vi "waypointVote.vi"() -> ()   [LabVIEW 2012]
panel:
  out "X of Center":dbl
  out "Y of Center":dbl
  out "XY Graph":cluster{dbl[], dbl[]}(graph)
  out "Radius":dbl
  in  "Boat Heading":dbl
  in  "Boat Pixel Y":dbl
  in  "Boat Pixel X":dbl
  in  "Desired Pixel Y":dbl
  in  "Desired Pixel X":dbl
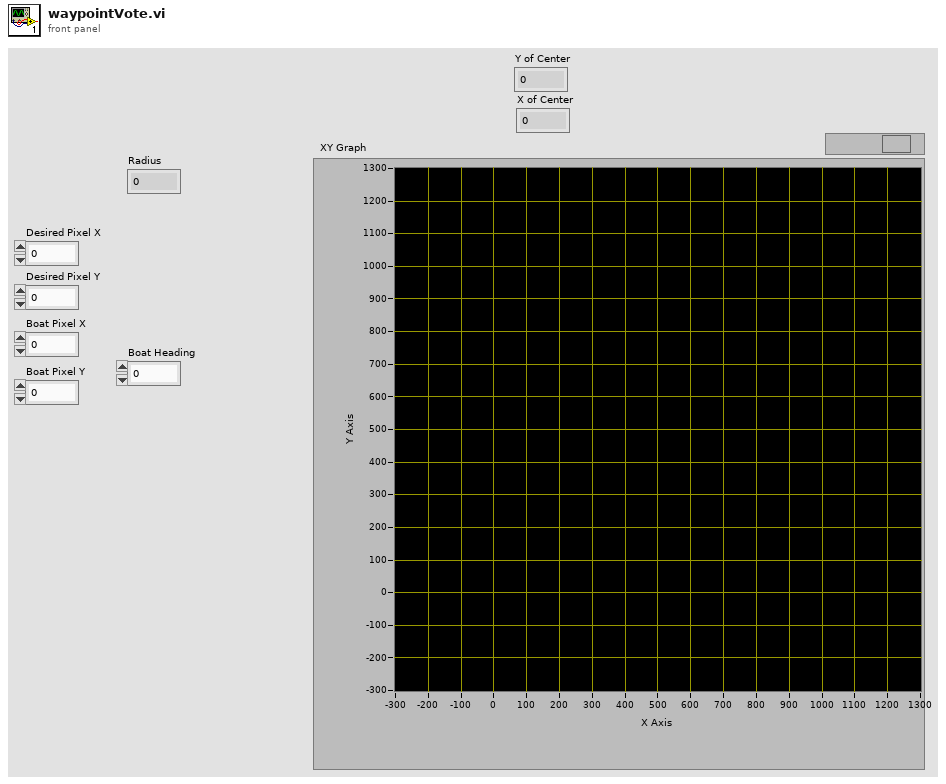
[diagram p1: front panel]
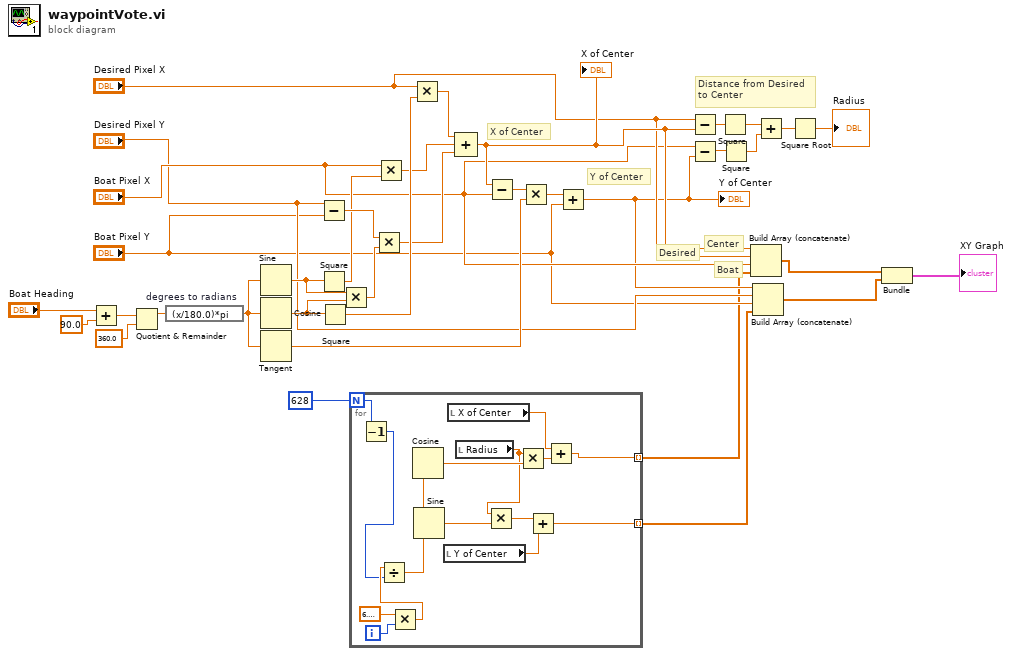
[diagram p0: block diagram]
diagram:
  # "Boat"
  # "Desired"
  # "Center"
  # "Distance from Desired\nto Center"
  # "Y of Center"
  # "X of Center"
  n1 = Add(x="Boat Heading", y=90.0) -> (x+y=w34:dbl)
  n2 = Quotient & Remainder(x=w34, y=360.0) -> (x-y*floor(x/y)=w8:dbl)  [unwired: 1 out]
  n3 = expression code="(x/180.0)*pi" "degrees to radians"(w8) -> (w7:dbl)
  n4 = Sine(x=w7) -> (sin(x)=w32:dbl)
  n5 = Cosine(x=w7) -> (cos(x)=w31:dbl)
  n6 = Tangent(1:w7) -> (0:w22:dbl)
  n7 = Subtract(x="Desired Pixel Y", y="Boat Pixel Y") -> (x-y=w30:dbl)
  n8 = Square(x=w32) -> (x^2=w28:dbl)
  n9 = Square(x=w31) -> (x^2=w27:dbl)
  n10 = Multiply(x=w32, y=w31) -> (x*y=w29:dbl)
  n11 = for {
    N: 628 -> [w40]
    tunnel: [w38] -> w3 mode=indexing
    tunnel: [w37] -> w4 mode=indexing
    i -> [w51]
    n12 = Decrement(x=w40) -> (x-1=w39:i32)
    n13 = Multiply(x=6.283185307179586, y=w51) -> (x*y=w41:dbl)
    n14 = Divide(x=w41, y=w39) -> (x/y=w50:dbl)
    n15 = Cosine(x=w50) -> (cos(x)=w49:dbl)
    n16 = Sine(x=w50) -> (sin(x)=w45:dbl)
    n17 = local read "Y of Center"() -> (w43:dbl)
    n18 = local read "X of Center"() -> (w47:dbl)
    n19 = local read "Radius"() -> (w46:dbl)
    n20 = Multiply(x=w46, y=w45) -> (x*y=w44:dbl)
    n21 = Multiply(x=w46, y=w49) -> (x*y=w48:dbl)
    n22 = Add(x=w44, y=w43) -> (x+y=w38:dbl)
    n23 = Add(x=w47, y=w48) -> (x+y=w37:dbl)
  }
  n24 = Multiply(x=w30, y=w29) -> (x*y=w25:dbl)
  n25 = Multiply(x="Boat Pixel X", y=w28) -> (x*y=w26:dbl)
  n26 = Multiply(x="Desired Pixel X", y=w27) -> (x*y=w24:dbl)
  n27 = Compound Arithmetic op=ADD(w24, w26, w25) -> (w14:dbl)
  "X of Center" <- w14
  n28 = Subtract(x=w14, y="Boat Pixel X") -> (x-y=w23:dbl)
  n29 = Multiply(x=w23, y=w22) -> (x*y=w21:dbl)
  n30 = Add(x=w21, y="Boat Pixel Y") -> (x+y=w11:dbl)
  "Y of Center" <- w11
  n31 = Subtract(x="Desired Pixel X", y=w14) -> (x-y=w18:dbl)
  n32 = Subtract(x="Boat Pixel X", y=w11) -> (x-y=w19:dbl)
  n33 = Square(x=w18) -> (x^2=w17:dbl)
  n34 = Square(x=w19) -> (x^2=w16:dbl)
  n35 = Build Array (concatenate)(w14, "Desired Pixel X", "Boat Pixel X", w4) -> (w2:dbl[])
  n36 = Build Array (concatenate)(w11, "Desired Pixel Y", "Boat Pixel Y", w3) -> (w1:dbl[])
  n37 = Add(x=w17, y=w16) -> (x+y=w20:dbl)
  n38 = Square Root(x=w20) -> (sqrt(x)=→"Radius":dbl)
  n39 = Bundle(w2, w1) -> (→"XY Graph":cluster{dbl[], dbl[]})  [unwired: 1 in]
